vi "Laser.vi"(8 "error in (no error)":errorcluster, 10 "Notifiers":T1, 11 "All Message Queue Cluster":T2) -> (0 "error out":errorcluster)   [LabVIEW 2017]
doc: "Ce VI est la partie visualisation du Laser"
uses:
  Lib QMH/AllMessageQueue Cluster.ctl
  Lib QMH/Message Cluster.ctl
  Lib Notifier/Notifier.ctl
  Laser UI data.ctl
  Laser config.ctl
  FGV Laser/Action Laser.ctl
  FGV Laser/FGV Laser Data.ctl
  PulsePickerValues.ctl
  Lib IHM Control/Front Panel Status.ctl
  support/Status.vi
  Lib QMH/MessageQueues.lvlib
  Lib IHM Control/IHM Control.lvlib
  Lib Notifier/Notifier.lvlib
panel:
  out "AOM Freq":dbl format="%#_3g"
  out "Amp Freq":dbl format="%#_3g"
  out "Connected":bool
  out "Status":string
  # "Laser"
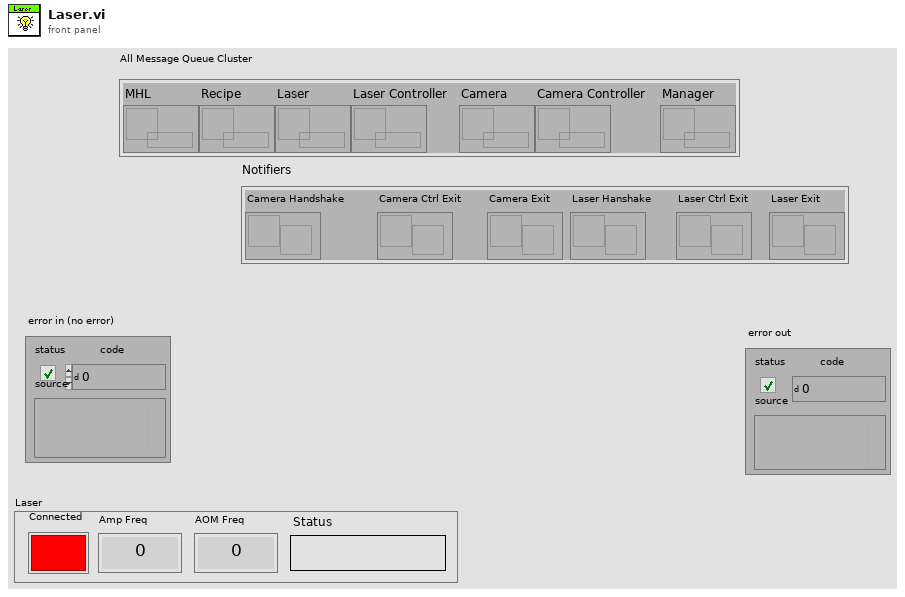
[diagram p1: front panel]
types:
  T1 = typedef "Notifier.lvlib/Notifier.ctl" = cluster{"Camera Handshake":refnum<notifier>, "Camera Ctrl Exit":refnum<notifier>, "Camera Exit":refnum<notifier>, "Laser Hanshake":refnum<notifier>, "Laser Ctrl Exit":refnum<notifier>, "Laser Exit":refnum<notifier>}
  T2 = typedef "MessageQueues.lvlib/AllMessageQueue Cluster.ctl" = cluster{"MHL":refnum<queue>, "Recipe":refnum<queue>, "Laser":refnum<queue>, "Laser Controller":refnum<queue>, "Camera":refnum<queue>, "Camera Controller":refnum<queue>, "Manager":refnum<queue>}
  T3 = typedef "FGV Laser Data.ctl" = cluster{"ONLINE":bool, "Power":dbl, "VISA resource name out":refnum<visa-resource-name>, "Time Out":dbl, "Status":string, "Read Count":u32, "On/OFF":bool, "Pulse Picker Set":T4}
  T4 = typedef "PulsePickerValues.ctl" = u16
  T5 = typedef "Action Laser.ctl" = enum16{"Initialize", "Connect", "Disconnect", "Set Power", "Get Power", "Set Pulse Picker", "Get Pulse Picker", "Laser ON", "Laser OFF", "Read Visa"}
  T6 = typedef "IHM Control.lvlib/Front Panel Status.ctl" = enum16{"Initialisation", "Enable Laser", "Enable Camera", "Disable Laser", "Disable Camera"}
  T7 = typedef "Laser config.ctl" = cluster{"VISA resource name":refnum<visa-resource-name>}
  T8 = typedef "Laser UI data.ctl" = cluster{"Connected":bool, "Status":string, "Power":dbl, "Pulse Picker":i32}
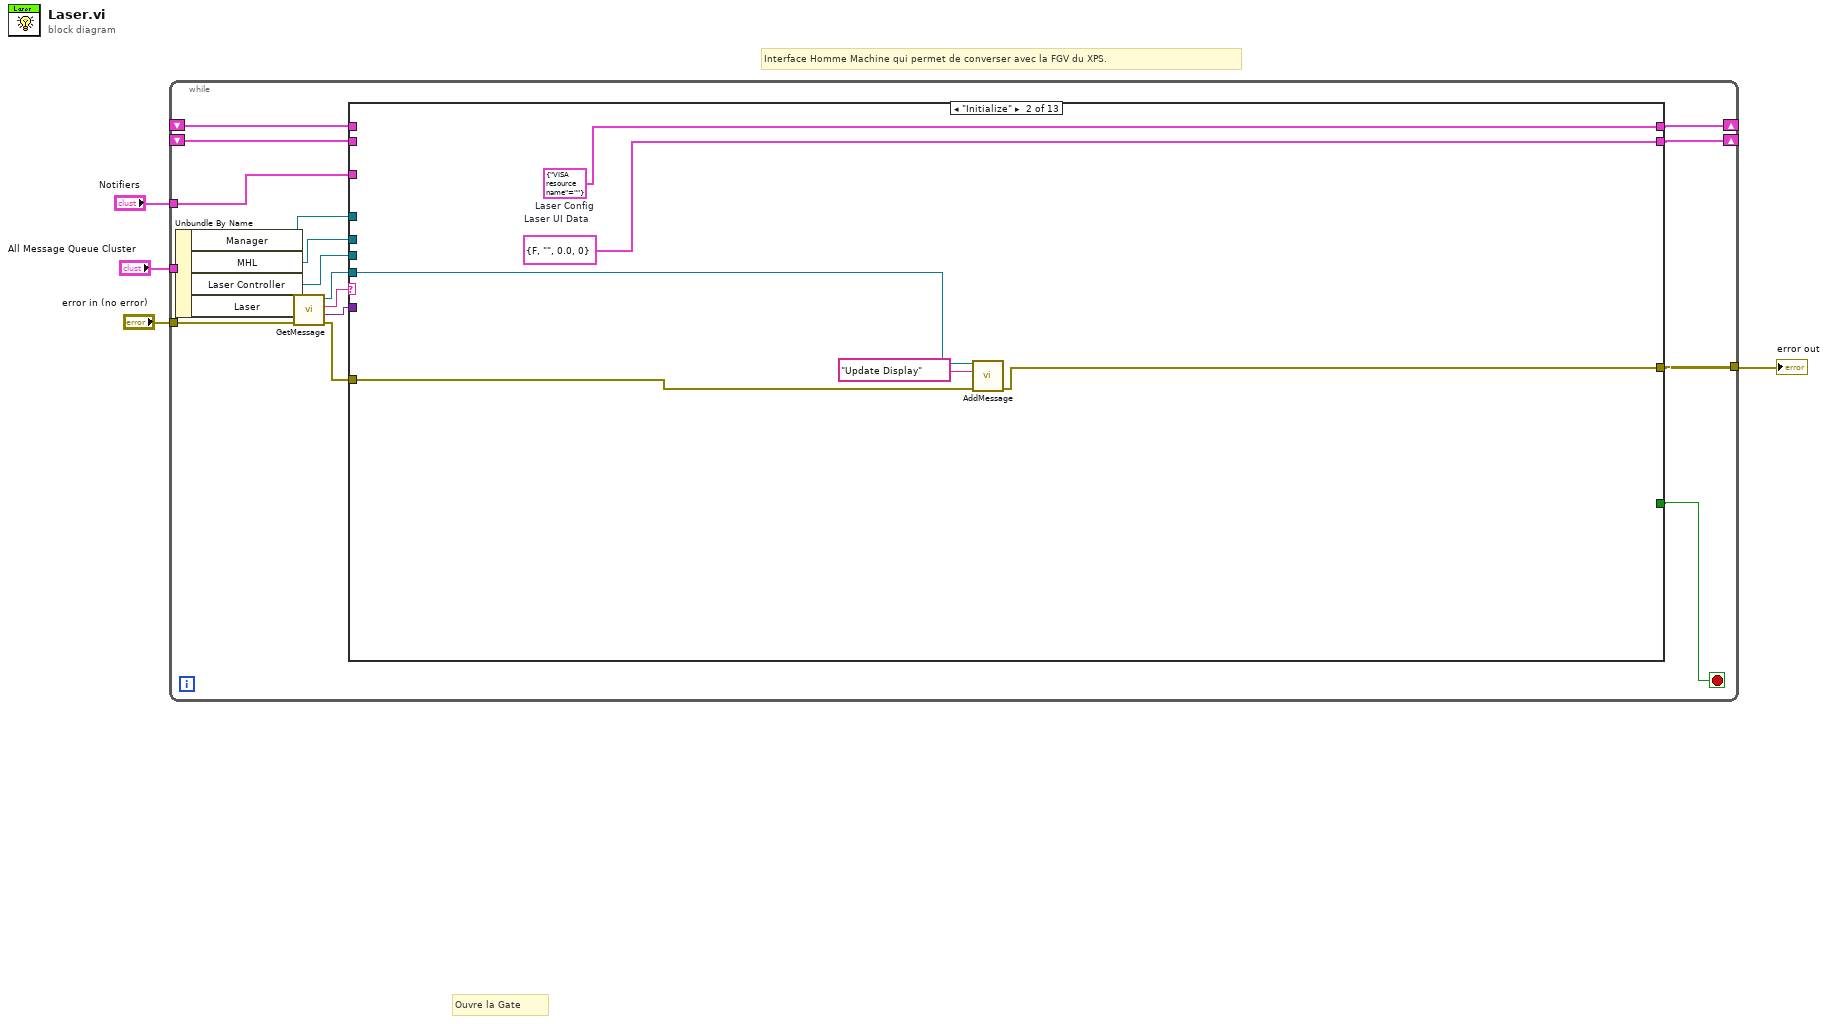
[diagram p0: block diagram]
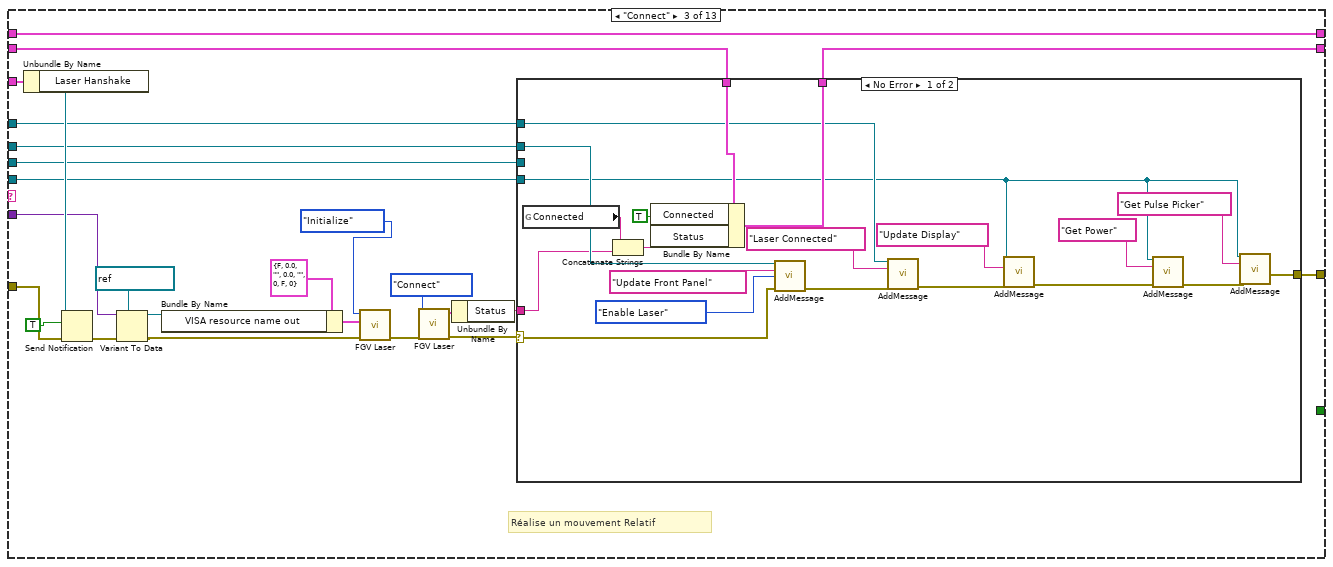
[diagram p3: hidden frame]
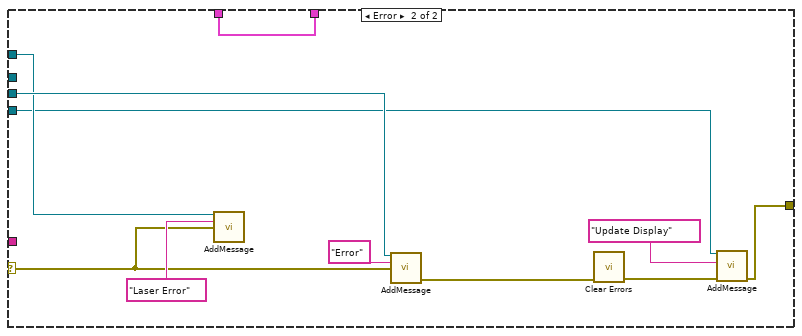
[diagram p4: hidden frame]
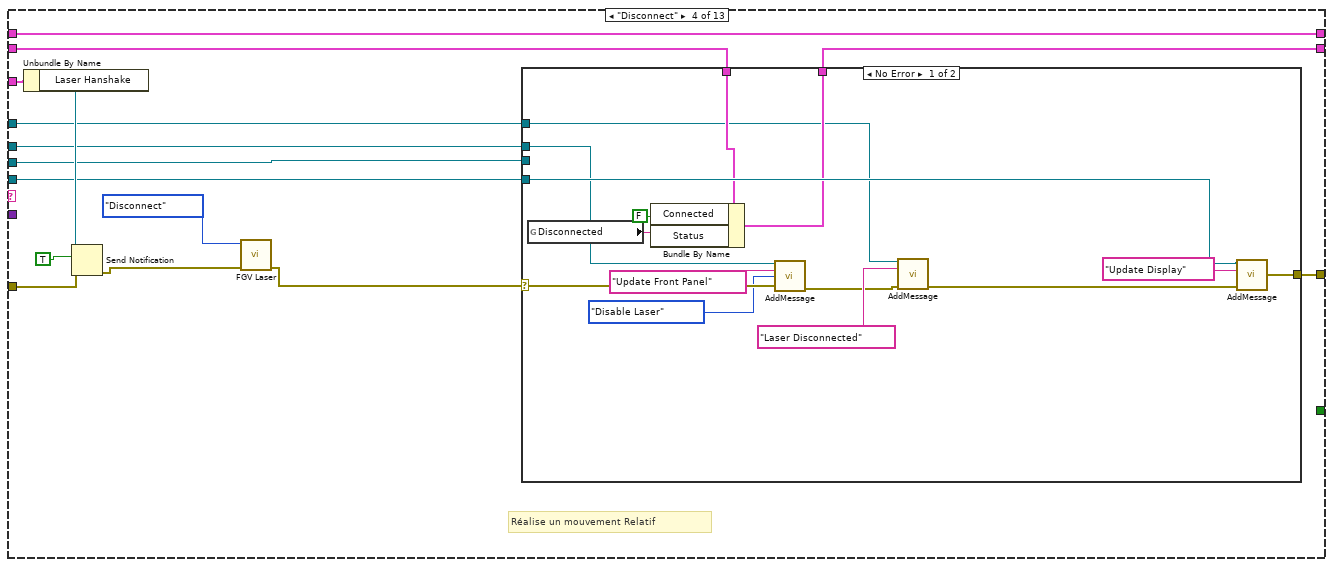
[diagram p5: hidden frame]
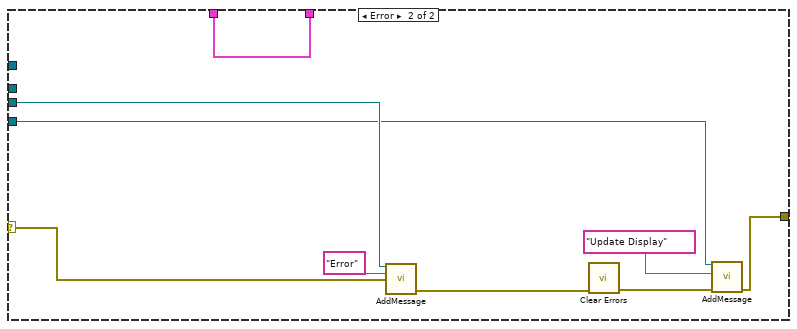
[diagram p6: hidden frame]
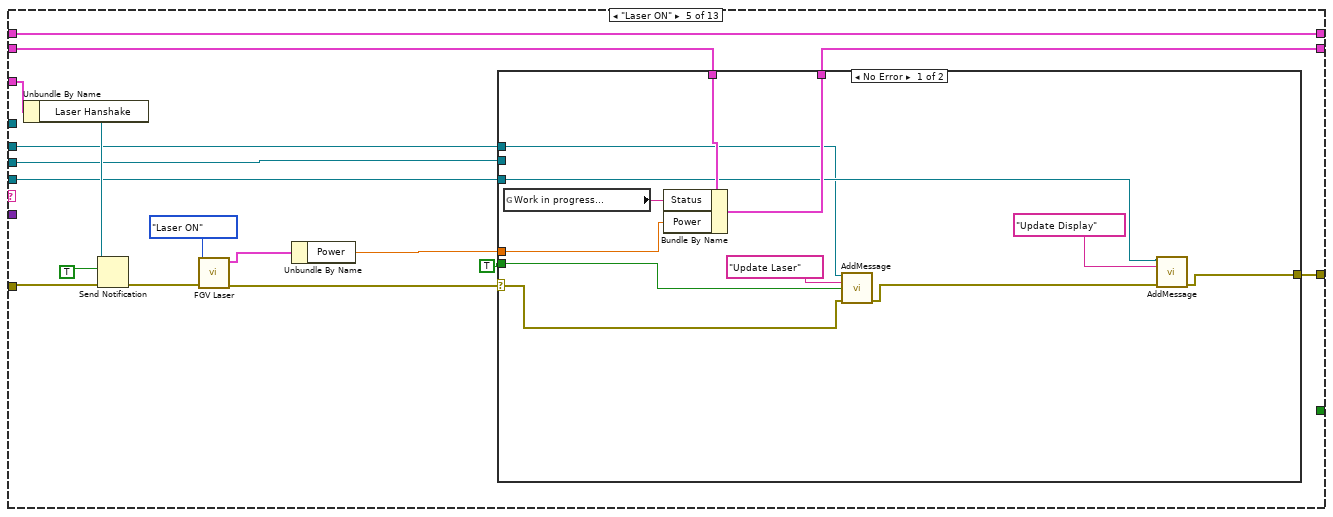
[diagram p7: hidden frame]
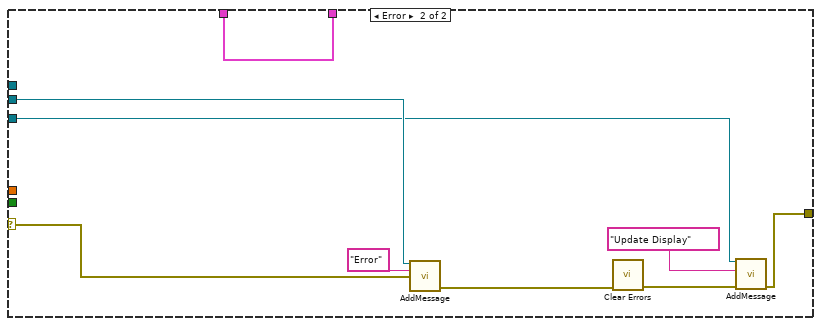
[diagram p8: hidden frame]
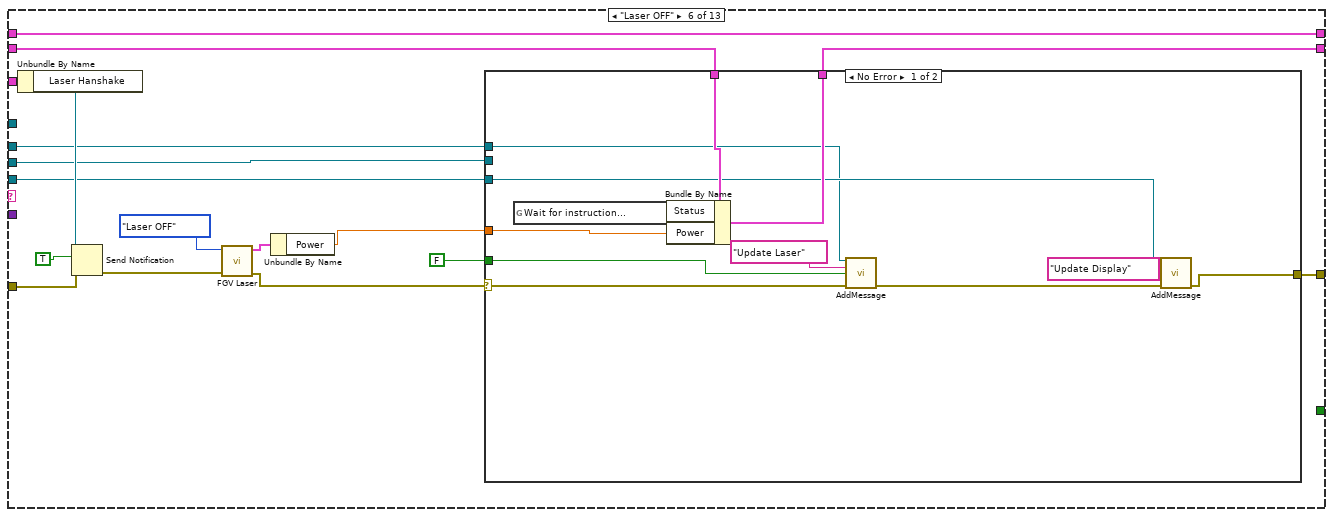
[diagram p9: hidden frame]
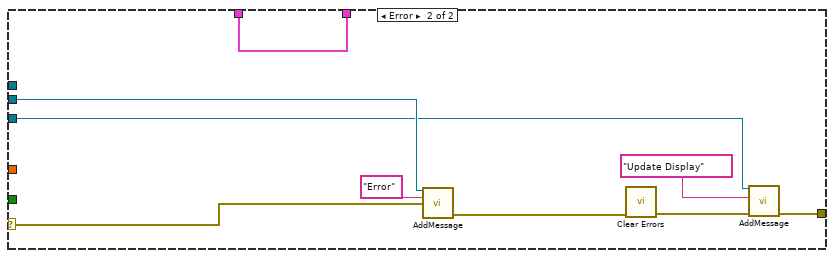
[diagram p10: hidden frame]
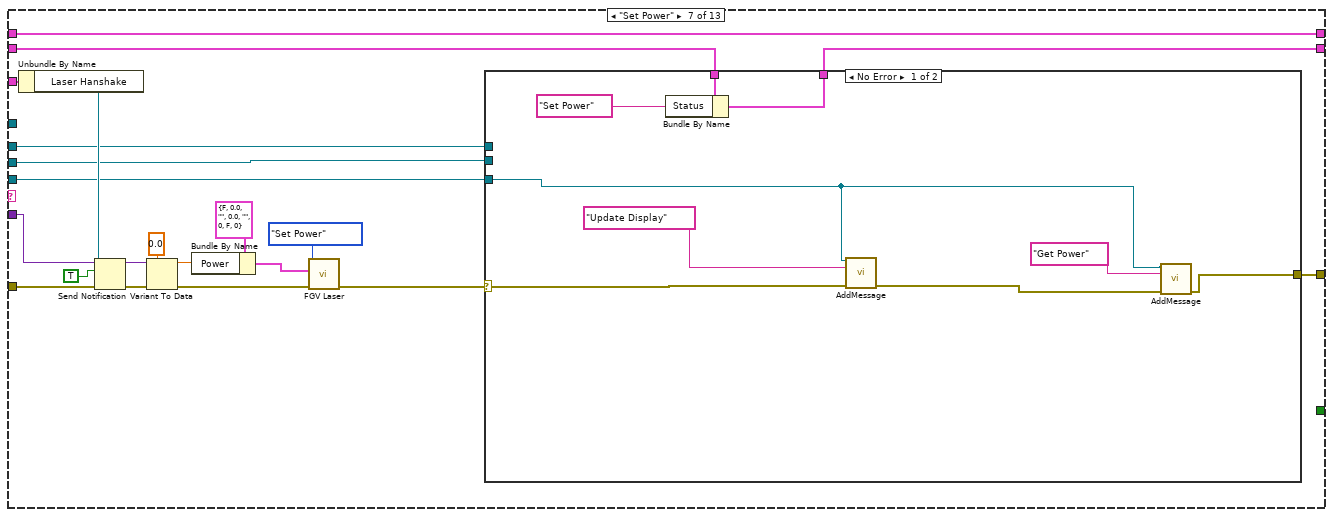
[diagram p11: hidden frame]
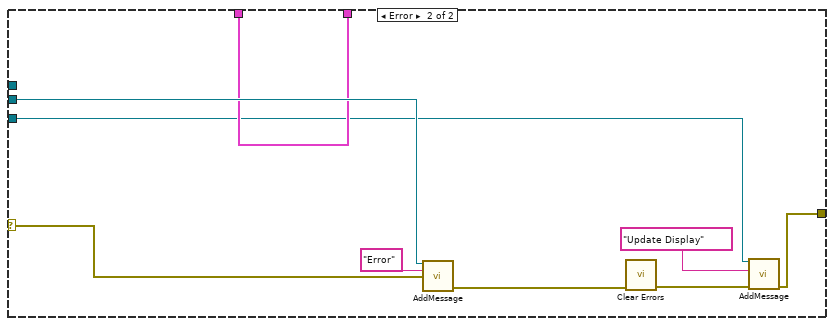
[diagram p12: hidden frame]
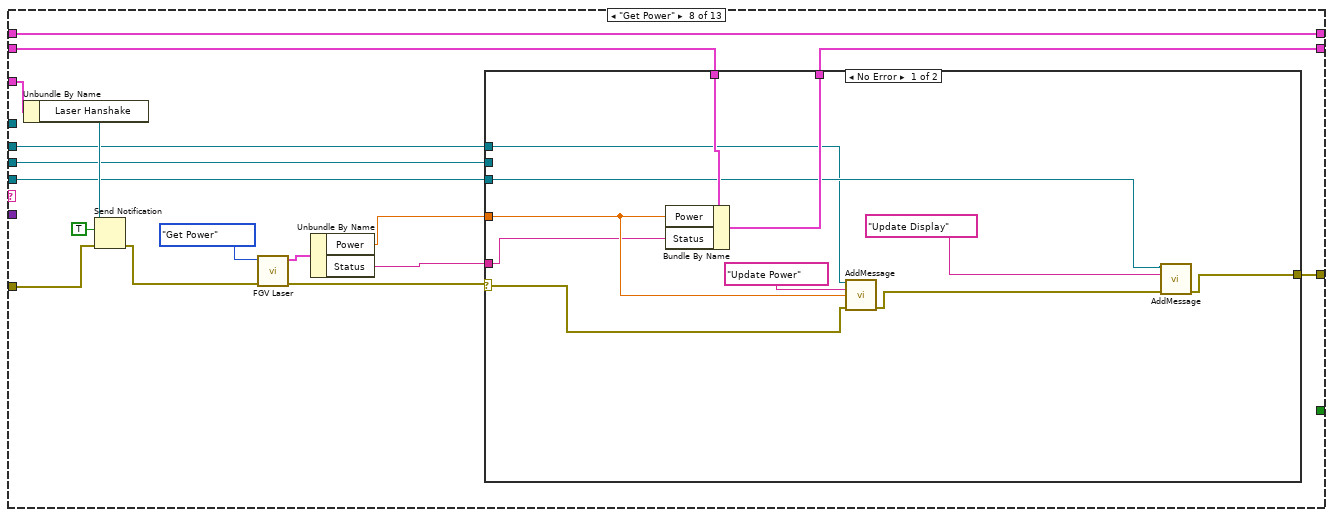
[diagram p13: hidden frame]
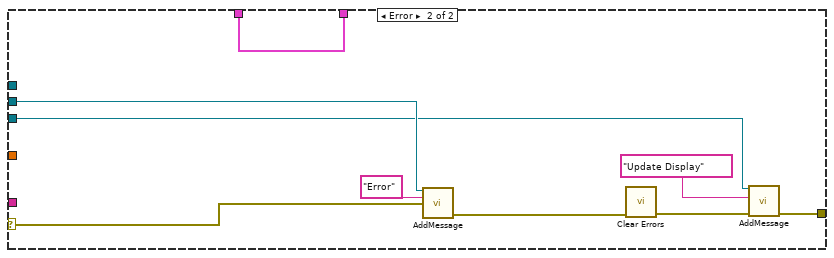
[diagram p14: hidden frame]
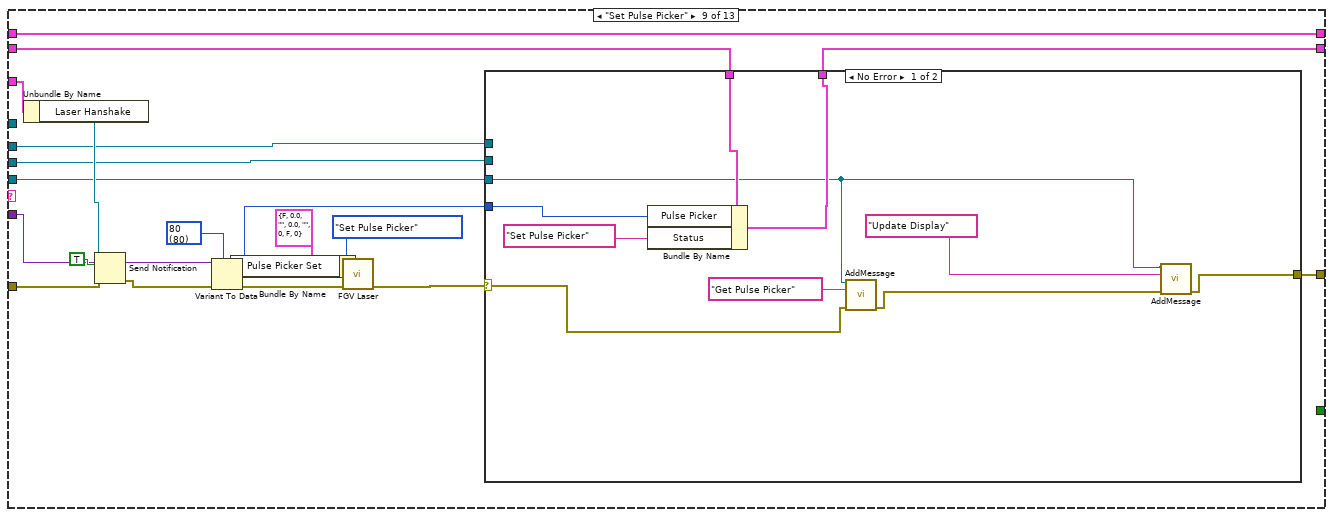
[diagram p15: hidden frame]
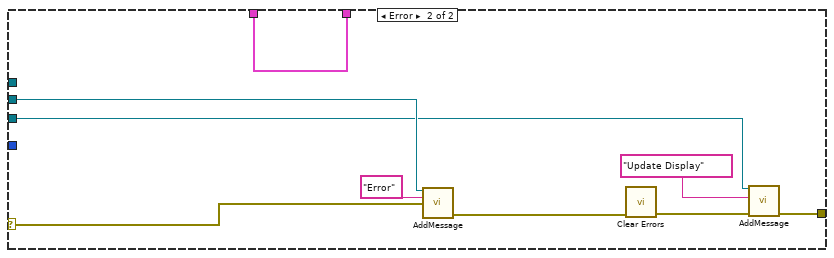
[diagram p16: hidden frame]
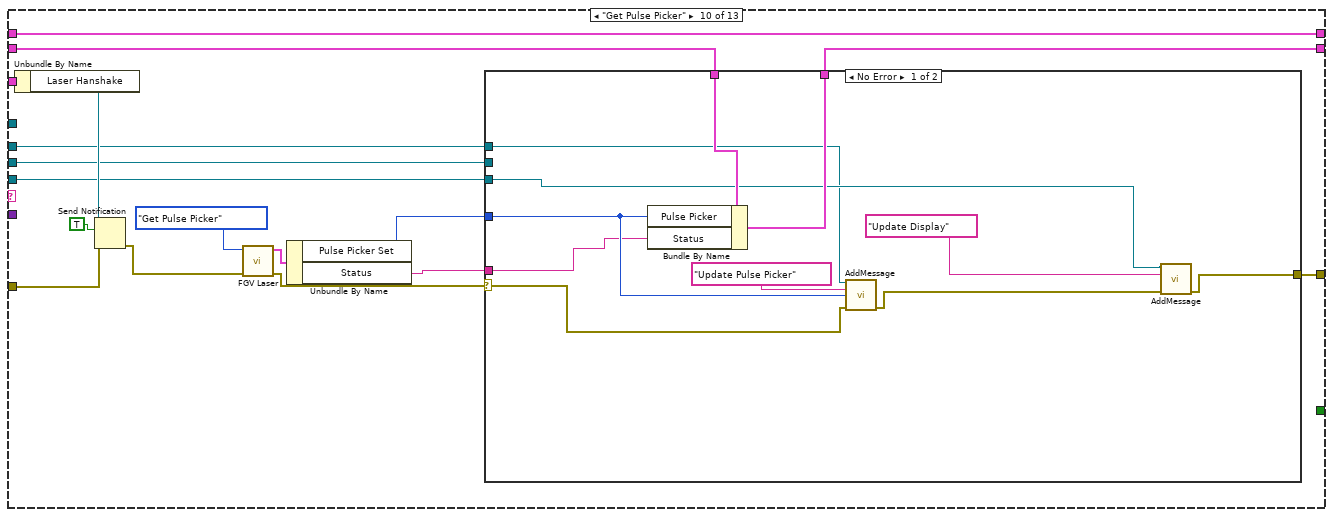
[diagram p17: hidden frame]
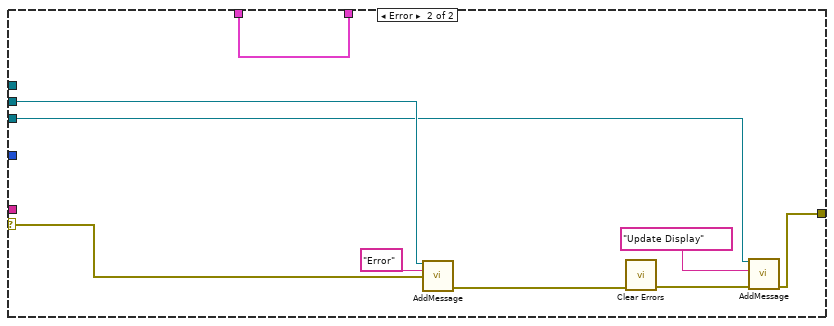
[diagram p18: hidden frame]
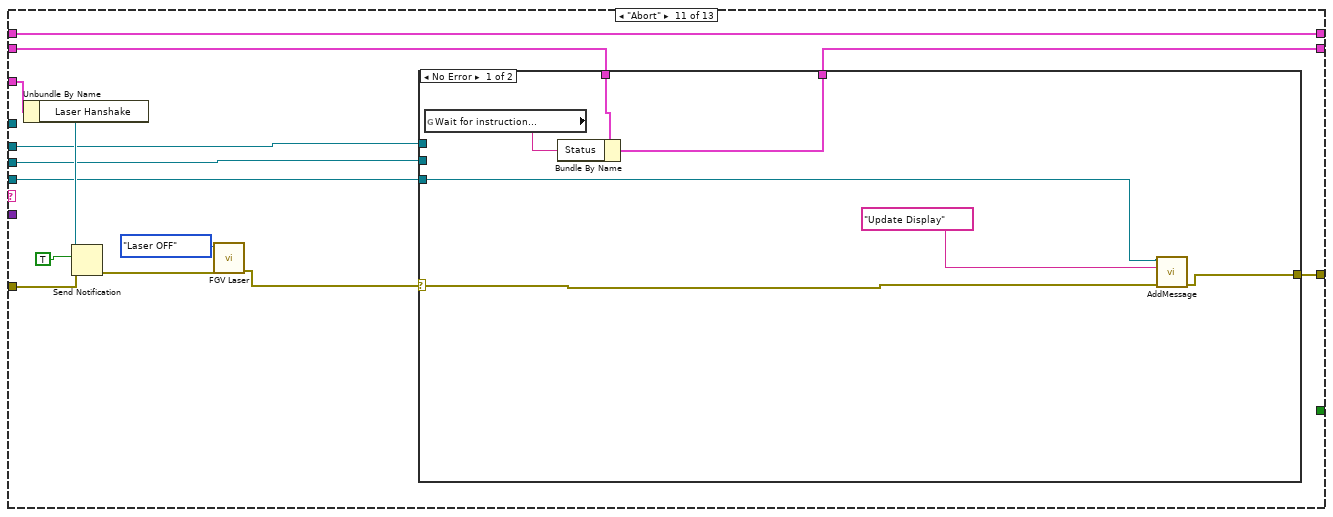
[diagram p19: hidden frame]
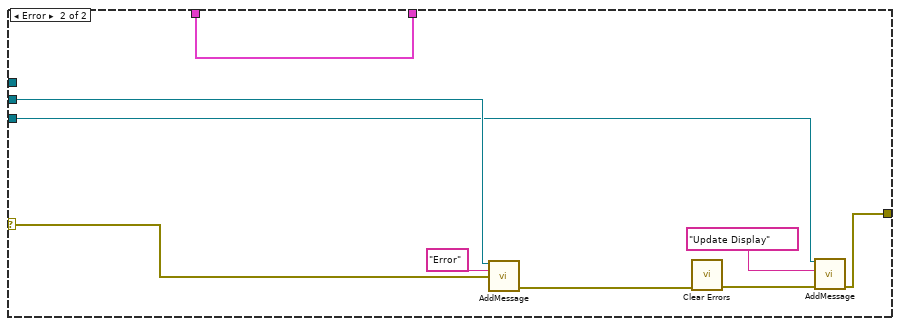
[diagram p20: hidden frame]
diagram:
  # "Interface Homme Machine qui permet de converser avec la FGV du XPS."
  # "Ouvre la Gate"
  n1 = while {
    tunnel: "All Message Queue Cluster" -> [w19]
    tunnel: "Notifiers" -> [w12]
    tunnel: "error in (no error)" -> [w20]
    tunnel: [w14] -> w1
    shift-right: [w16] -> _
    shift-left: _ -> [w18]
    shift-right: [w15] -> _
    shift-left: _ -> [w17]
    stop <- w13 stop-if-true
    n2 = Unbundle By Name(w19) -> ("Manager"=w11:refnum<queue>, "MHL"=w10:refnum<queue>, "Laser Controller"=w9:refnum<queue>, "Laser"=w21:refnum<queue>)
    n3 = call "GetMessage.vi"("entrée d'erreur"=w20, "Message queue"=w21) -> ("sortie d'erreur"=w7:errorcluster, "Data"=w6:variant, "Message"=w5:string, "Dup Message Queue"=w8:refnum<queue>)  [unwired: 6 in]
    n4 = case shown="\"Initialize\"" w5 {
      tunnel: w12 -> [_ _ w53 w100 w141 w179 w220 w255 w295 w331 w365 _ w400]
      tunnel: w8 -> [_ w27 w52 w99 w140 w178 w219 w254 w294 w330 w364 _ w394]
      tunnel: w6 -> [_ _ w42 _ _ _ w212 _ w287 _ _ _ _]
      tunnel: w7 -> [w24 w29 w46 w93 w135 w173 w210 w247 w286 w323 w359 w389 w395]
      tunnel: [w24 w28 w51 w98 w139 w177 w218 w253 w293 w329 w363 w389 w397] -> w14
      tunnel: w9 -> [_ _ w50 w97 w138 w176 w217 w252 w292 w328 w362 _ _]
      tunnel: [_ _ _ _ _ _ _ _ _ _ _ _ TRUE] -> w13
      tunnel: w18 -> [w23 _ w49 w96 w137 w175 w216 w251 w291 w327 w361 w390 w396]
      tunnel: [w23 w26 w49 w96 w137 w175 w216 w251 w291 w327 w361 w390 w396] -> w16
      tunnel: w17 -> [w22 _ w48 w95 w133 w171 w213 w248 w288 w324 w357 w388 w393]
      tunnel: [w22 w25 w47 w94 w136 w174 w215 w250 w290 w326 w360 w388 w393] -> w15
      tunnel: w10 -> [_ _ w45 w92 w134 w172 w214 w249 w289 w325 w358 _ _]
      tunnel: w11 -> [_ _ w44 w91 _ _ _ _ _ _ _ _ _]
      frame Default {
        # "ne fait rien si le message dépilé n'existe pas"
      }
      frame "Initialize" {
        w26 = T7 {"VISA resource name"=""}  # Laser Config
        w25 = T8 {"Connected"=FALSE, "Status"="", "Power"=0.0, "Pulse Picker"=0}  # Laser UI Data
        n5 = call "AddMessage.vi"("Message queue"=w27, "Message"="Update Display", "entrée d'erreur (pas d'erreur)"=w29) -> ("error out"=w28:errorcluster)  [unwired: 11 in, 1 out]
      }
      frame "Connect" {
        # "Réalise un mouvement Relatif"
        n6 = Unbundle By Name(w53) -> ("Laser Hanshake"=w55:refnum<notifier>)
        n7 = Send Notification(notification=TRUE, notifier=w55, error in (no error)=w46) -> (error out=w43:errorcluster)  [unwired: 1 out]
        n8 = Variant To Data(error in=w43, type=refnum<visa-resource-name> "COM30" ("VISA resource name out"), Variant=w42) -> (data=w36:refnum<visa-resource-name>, error out=w35:errorcluster)
        n9 = Bundle By Name(cluster=T3 {"ONLINE"=FALSE, "Power"=0.0, "VISA resource name out"="", "Time Out"=0.0, "Status"="", "Read Count"=0, "On/OFF"=FALSE, "Pulse Picker Set"=0} ("FGV Laser Data In"), "VISA resource name out"=w36) -> (w37:T3)
        n10 = call "FGV Laser.vi"("error in (no error)"=w35, "FGV Laser Data In"=w37, "Action"=Action_Laser."Initialize") -> ("error out"=w39:errorcluster)  [unwired: 7 in, 1 out]
        n11 = call "FGV Laser.vi"("error in (no error)"=w39, "Action"=Action_Laser."Connect") -> ("error out"=w33:errorcluster, "FGV Laser Data Out"=w32:T3)  [unwired: 8 in]
        n12 = Unbundle By Name(w32) -> ("Status"=w31:string)
        n13 = case shown="No Error" w33 {
          selector: w33 -> [w72 w78]
          tunnel: w52 -> [w57 w77]
          tunnel: [w59 w83] -> w51
          tunnel: w50 -> [_ w82]
          tunnel: w48 -> [w75 w81]
          tunnel: [w74 w81] -> w47
          tunnel: w45 -> [w71 _]
          tunnel: w44 -> [w66 w79]
          tunnel: w31 -> [w62 _]
          frame No Error {
            n14 = global read "Status.vi" "Connected"() -> (w64:string)
            n15 = Concatenate Strings(w64, w62) -> (w63:string)
            n16 = Bundle By Name(cluster=w75, "Connected"=TRUE, "Status"=w63) -> (w74:T8)
            n17 = call "AddMessage.vi"("Message queue"=w71, "Message"="Update Front Panel", "Data"=Front_Panel_Status."Enable Laser" ("Front Panel status"), "entrée d'erreur (pas d'erreur)"=w72) -> ("error out"=w68:errorcluster)  [unwired: 10 in, 1 out]
            n18 = call "AddMessage.vi"("Message queue"=w66, "Message"="Laser Connected", "entrée d'erreur (pas d'erreur)"=w68) -> ("error out"=w67:errorcluster)  [unwired: 11 in, 1 out]
            n19 = call "AddMessage.vi"("Message queue"=w57, "Message"="Update Display", "entrée d'erreur (pas d'erreur)"=w67) -> ("error out"=w61:errorcluster)  [unwired: 11 in, 1 out]
            n20 = call "AddMessage.vi"("Message queue"=w57, "Message"="Get Power", "entrée d'erreur (pas d'erreur)"=w61) -> ("error out"=w60:errorcluster)  [unwired: 11 in, 1 out]
            n21 = call "AddMessage.vi"("Message queue"=w57, "Message"="Get Pulse Picker", "entrée d'erreur (pas d'erreur)"=w60) -> ("error out"=w59:errorcluster)  [unwired: 11 in, 1 out]
          }
          frame Error {
            n22 = call "AddMessage.vi"("Message queue"=w79, "Message"="Laser Error", "Data"=w78) -> ()  [unwired: 11 in, 2 out]
            n23 = call "AddMessage.vi"("Message queue"=w82, "Message"="Error", "Data"=w78) -> ("error out"=w86:errorcluster)  [unwired: 11 in, 1 out]
            n24 = call <vilib>:"Clear Errors.vi"("error in (no error)"=w86) -> ("error out"=w84:errorcluster)  [unwired: 5 in, 1 out]
            n25 = call "AddMessage.vi"("Message queue"=w77, "Message"="Update Display", "entrée d'erreur (pas d'erreur)"=w84) -> ("error out"=w83:errorcluster)  [unwired: 11 in, 1 out]
          }
        }
      }
      frame "Disconnect" {
        # "Réalise un mouvement Relatif"
        n26 = Unbundle By Name(w100) -> ("Laser Hanshake"=w102:refnum<notifier>)
        n27 = Send Notification(notification=TRUE, notifier=w102, error in (no error)=w93) -> (error out=w90:errorcluster)  [unwired: 1 out]
        n28 = call "FGV Laser.vi"("error in (no error)"=w90, "Action"=Action_Laser."Disconnect") -> ("error out"=w89:errorcluster)  [unwired: 8 in, 1 out]
        n29 = case shown="No Error" w89 {
          selector: w89 -> [w111 w121]
          tunnel: w99 -> [w117 w118]
          tunnel: [w115 w122] -> w98
          tunnel: w97 -> [_ w120]
          tunnel: w95 -> [w114 w119]
          tunnel: [w113 w119] -> w94
          tunnel: w92 -> [w110 _]
          tunnel: w91 -> [w104 _]
          frame No Error {
            n30 = global read "Status.vi" "Disconnected"() -> (w103:string)
            n31 = Bundle By Name(cluster=w114, "Connected"=FALSE, "Status"=w103) -> (w113:T8)
            n32 = call "AddMessage.vi"("Message queue"=w110, "Message"="Update Front Panel", "Data"=Front_Panel_Status."Disable Laser" ("Front Panel status"), "entrée d'erreur (pas d'erreur)"=w111) -> ("error out"=w106:errorcluster)  [unwired: 10 in, 1 out]
            n33 = call "AddMessage.vi"("Message queue"=w104, "Message"="Laser Disconnected", "entrée d'erreur (pas d'erreur)"=w106) -> ("error out"=w105:errorcluster)  [unwired: 11 in, 1 out]
            n34 = call "AddMessage.vi"("Message queue"=w117, "Message"="Update Display", "entrée d'erreur (pas d'erreur)"=w105) -> ("error out"=w115:errorcluster)  [unwired: 11 in, 1 out]
          }
          frame Error {
            n35 = call "AddMessage.vi"("Message queue"=w120, "Message"="Error", "Data"=w121) -> ("error out"=w125:errorcluster)  [unwired: 11 in, 1 out]
            n36 = call <vilib>:"Clear Errors.vi"("error in (no error)"=w125) -> ("error out"=w123:errorcluster)  [unwired: 5 in, 1 out]
            n37 = call "AddMessage.vi"("Message queue"=w118, "Message"="Update Display", "entrée d'erreur (pas d'erreur)"=w123) -> ("error out"=w122:errorcluster)  [unwired: 11 in, 1 out]
          }
        }
      }
      frame "Laser ON" {
        n38 = Unbundle By Name(w141) -> ("Laser Hanshake"=w143:refnum<notifier>)
        n39 = Send Notification(notification=TRUE, notifier=w143, error in (no error)=w135) -> (error out=w131:errorcluster)  [unwired: 1 out]
        n40 = call "FGV Laser.vi"("error in (no error)"=w131, "Action"=Action_Laser."Laser ON") -> ("error out"=w130:errorcluster, "FGV Laser Data Out"=w128:T3)  [unwired: 8 in]
        n41 = Unbundle By Name(w128) -> ("Power"=w127:dbl)
        n42 = case shown="No Error" w130 {
          selector: w130 -> [w151 w159]
          tunnel: w140 -> [w152 w156]
          tunnel: [w146 w160] -> w139
          tunnel: w138 -> [_ w158]
          tunnel: w133 -> [w154 w157]
          tunnel: [w153 w157] -> w136
          tunnel: w134 -> [w149 _]
          tunnel: TRUE -> [w145 _]
          tunnel: w127 -> [w144 _]
          frame No Error {
            n43 = global read "Status.vi" "Work in progress..."() -> (w147:string)
            n44 = Bundle By Name(cluster=w154, "Status"=w147, "Power"=w144) -> (w153:T8)
            n45 = call "AddMessage.vi"("Message queue"=w149, "Message"="Update Laser", "Data"=w145, "entrée d'erreur (pas d'erreur)"=w151) -> ("error out"=w150:errorcluster)  [unwired: 10 in, 1 out]
            n46 = call "AddMessage.vi"("Message queue"=w152, "Message"="Update Display", "entrée d'erreur (pas d'erreur)"=w150) -> ("error out"=w146:errorcluster)  [unwired: 11 in, 1 out]
          }
          frame Error {
            n47 = call "AddMessage.vi"("Message queue"=w158, "Message"="Error", "Data"=w159) -> ("error out"=w163:errorcluster)  [unwired: 11 in, 1 out]
            n48 = call <vilib>:"Clear Errors.vi"("error in (no error)"=w163) -> ("error out"=w161:errorcluster)  [unwired: 5 in, 1 out]
            n49 = call "AddMessage.vi"("Message queue"=w156, "Message"="Update Display", "entrée d'erreur (pas d'erreur)"=w161) -> ("error out"=w160:errorcluster)  [unwired: 11 in, 1 out]
          }
        }
      }
      frame "Laser OFF" {
        n50 = Unbundle By Name(w179) -> ("Laser Hanshake"=w181:refnum<notifier>)
        n51 = Send Notification(notification=TRUE, notifier=w181, error in (no error)=w173) -> (error out=w169:errorcluster)  [unwired: 1 out]
        n52 = call "FGV Laser.vi"("error in (no error)"=w169, "Action"=Action_Laser."Laser OFF") -> ("error out"=w168:errorcluster, "FGV Laser Data Out"=w166:T3)  [unwired: 8 in]
        n53 = Unbundle By Name(w166) -> ("Power"=w165:dbl)
        n54 = case shown="No Error" w168 {
          selector: w168 -> [w183 w197]
          tunnel: w178 -> [w187 w194]
          tunnel: [w184 w198] -> w177
          tunnel: w176 -> [_ w196]
          tunnel: w171 -> [w189 w195]
          tunnel: [w188 w195] -> w174
          tunnel: w172 -> [w186 _]
          tunnel: FALSE -> [w185 _]
          tunnel: w165 -> [w182 _]
          frame No Error {
            n55 = global read "Status.vi" "Wait for instruction..."() -> (w190:string)
            n56 = Bundle By Name(cluster=w189, "Status"=w190, "Power"=w182) -> (w188:T8)
            n57 = call "AddMessage.vi"("Message queue"=w186, "Message"="Update Laser", "Data"=w185, "entrée d'erreur (pas d'erreur)"=w183) -> ("error out"=w192:errorcluster)  [unwired: 10 in, 1 out]
            n58 = call "AddMessage.vi"("Message queue"=w187, "Message"="Update Display", "entrée d'erreur (pas d'erreur)"=w192) -> ("error out"=w184:errorcluster)  [unwired: 11 in, 1 out]
          }
          frame Error {
            n59 = call "AddMessage.vi"("Message queue"=w196, "Message"="Error", "Data"=w197) -> ("error out"=w201:errorcluster)  [unwired: 11 in, 1 out]
            n60 = call <vilib>:"Clear Errors.vi"("error in (no error)"=w201) -> ("error out"=w199:errorcluster)  [unwired: 5 in, 1 out]
            n61 = call "AddMessage.vi"("Message queue"=w194, "Message"="Update Display", "entrée d'erreur (pas d'erreur)"=w199) -> ("error out"=w198:errorcluster)  [unwired: 11 in, 1 out]
          }
        }
      }
      frame "Set Power" {
        n62 = Unbundle By Name(w220) -> ("Laser Hanshake"=w222:refnum<notifier>)
        n63 = Send Notification(notification=TRUE, notifier=w222, error in (no error)=w210) -> (error out=w209:errorcluster)  [unwired: 1 out]
        n64 = Variant To Data(error in=w209, type=0.0, Variant=w212) -> (data=w207:dbl, error out=w205:errorcluster)
        n65 = Bundle By Name(cluster=T3 {"ONLINE"=FALSE, "Power"=0.0, "VISA resource name out"="", "Time Out"=0.0, "Status"="", "Read Count"=0, "On/OFF"=FALSE, "Pulse Picker Set"=0} ("FGV Laser Data In"), "Power"=w207) -> (w206:T3)
        n66 = call "FGV Laser.vi"("error in (no error)"=w205, "FGV Laser Data In"=w206, "Action"=Action_Laser."Set Power") -> ("error out"=w204:errorcluster)  [unwired: 7 in, 1 out]
        n67 = case shown="No Error" w204 {
          selector: w204 -> [w228 w235]
          tunnel: w219 -> [w225 w232]
          tunnel: [w227 w236] -> w218
          tunnel: w217 -> [_ w234]
          tunnel: w213 -> [w230 w233]
          tunnel: [w229 w233] -> w215
          tunnel: w214 -> [_ _]
          frame No Error {
            n68 = Bundle By Name(cluster=w230, "Status"="Set Power") -> (w229:T8)
            n69 = call "AddMessage.vi"("Message queue"=w225, "Message"="Update Display", "entrée d'erreur (pas d'erreur)"=w228) -> ("error out"=w231:errorcluster)  [unwired: 11 in, 1 out]
            n70 = call "AddMessage.vi"("Message queue"=w225, "Message"="Get Power", "entrée d'erreur (pas d'erreur)"=w231) -> ("error out"=w227:errorcluster)  [unwired: 11 in, 1 out]
          }
          frame Error {
            n71 = call "AddMessage.vi"("Message queue"=w234, "Message"="Error", "Data"=w235) -> ("error out"=w239:errorcluster)  [unwired: 11 in, 1 out]
            n72 = call <vilib>:"Clear Errors.vi"("error in (no error)"=w239) -> ("error out"=w237:errorcluster)  [unwired: 5 in, 1 out]
            n73 = call "AddMessage.vi"("Message queue"=w232, "Message"="Update Display", "entrée d'erreur (pas d'erreur)"=w237) -> ("error out"=w236:errorcluster)  [unwired: 11 in, 1 out]
          }
        }
      }
      frame "Get Power" {
        n74 = Unbundle By Name(w255) -> ("Laser Hanshake"=w257:refnum<notifier>)
        n75 = Send Notification(notification=TRUE, notifier=w257, error in (no error)=w247) -> (error out=w246:errorcluster)  [unwired: 1 out]
        n76 = call "FGV Laser.vi"("error in (no error)"=w246, "Action"=Action_Laser."Get Power") -> ("error out"=w245:errorcluster, "FGV Laser Data Out"=w243:T3)  [unwired: 8 in]
        n77 = Unbundle By Name(w243) -> ("Power"=w242:dbl, "Status"=w241:string)
        n78 = case shown="No Error" w245 {
          selector: w245 -> [w263 w272]
          tunnel: w254 -> [w261 w269]
          tunnel: [w262 w273] -> w253
          tunnel: w252 -> [_ w271]
          tunnel: w248 -> [w265 w270]
          tunnel: [w264 w270] -> w250
          tunnel: w249 -> [w260 _]
          tunnel: w242 -> [w259 _]
          tunnel: w241 -> [w258 _]
          frame No Error {
            n79 = Bundle By Name(cluster=w265, "Power"=w259, "Status"=w258) -> (w264:T8)
            n80 = call "AddMessage.vi"("Message queue"=w260, "Message"="Update Power", "Data"=w259, "entrée d'erreur (pas d'erreur)"=w263) -> ("error out"=w267:errorcluster)  [unwired: 10 in, 1 out]
            n81 = call "AddMessage.vi"("Message queue"=w261, "Message"="Update Display", "entrée d'erreur (pas d'erreur)"=w267) -> ("error out"=w262:errorcluster)  [unwired: 11 in, 1 out]
          }
          frame Error {
            n82 = call "AddMessage.vi"("Message queue"=w271, "Message"="Error", "Data"=w272) -> ("error out"=w276:errorcluster)  [unwired: 11 in, 1 out]
            n83 = call <vilib>:"Clear Errors.vi"("error in (no error)"=w276) -> ("error out"=w274:errorcluster)  [unwired: 5 in, 1 out]
            n84 = call "AddMessage.vi"("Message queue"=w269, "Message"="Update Display", "entrée d'erreur (pas d'erreur)"=w274) -> ("error out"=w273:errorcluster)  [unwired: 11 in, 1 out]
          }
        }
      }
      frame "Set Pulse Picker" {
        w278 = u16 80 items=["80"=80, "40"=40, "20"=20] ("Pulse Picker Set")
        n85 = Unbundle By Name(w295) -> ("Laser Hanshake"=w297:refnum<notifier>)
        n86 = Send Notification(notification=TRUE, notifier=w297, error in (no error)=w286) -> (error out=w285:errorcluster)  [unwired: 1 out]
        n87 = Variant To Data(error in=w285, type=w278, Variant=w287) -> (data=w279:u16, error out=w284:errorcluster)
        n88 = Bundle By Name(cluster=T3 {"ONLINE"=FALSE, "Power"=0.0, "VISA resource name out"="", "Time Out"=0.0, "Status"="", "Read Count"=0, "On/OFF"=FALSE, "Pulse Picker Set"=0} ("FGV Laser Data In"), "Pulse Picker Set"=w279) -> (w281:T3)
        n89 = call "FGV Laser.vi"("error in (no error)"=w284, "FGV Laser Data In"=w281, "Action"=Action_Laser."Set Pulse Picker") -> ("error out"=w283:errorcluster)  [unwired: 7 in, 1 out]
        n90 = case shown="No Error" w283 {
          selector: w283 -> [w302 w311]
          tunnel: w294 -> [w299 w308]
          tunnel: [w301 w312] -> w293
          tunnel: w292 -> [_ w310]
          tunnel: w288 -> [w304 w309]
          tunnel: [w303 w309] -> w290
          tunnel: w289 -> [_ _]
          tunnel: w279 -> [w298 _]
          frame No Error {
            n91 = Bundle By Name(cluster=w304, "Pulse Picker"=w298, "Status"="Set Pulse Picker") -> (w303:T8)
            n92 = call "AddMessage.vi"("Message queue"=w299, "Message"="Get Pulse Picker", "entrée d'erreur (pas d'erreur)"=w302) -> ("error out"=w306:errorcluster)  [unwired: 11 in, 1 out]
            n93 = call "AddMessage.vi"("Message queue"=w299, "Message"="Update Display", "entrée d'erreur (pas d'erreur)"=w306) -> ("error out"=w301:errorcluster)  [unwired: 11 in, 1 out]
          }
          frame Error {
            n94 = call "AddMessage.vi"("Message queue"=w310, "Message"="Error", "Data"=w311) -> ("error out"=w315:errorcluster)  [unwired: 11 in, 1 out]
            n95 = call <vilib>:"Clear Errors.vi"("error in (no error)"=w315) -> ("error out"=w313:errorcluster)  [unwired: 5 in, 1 out]
            n96 = call "AddMessage.vi"("Message queue"=w308, "Message"="Update Display", "entrée d'erreur (pas d'erreur)"=w313) -> ("error out"=w312:errorcluster)  [unwired: 11 in, 1 out]
          }
        }
      }
      frame "Get Pulse Picker" {
        n97 = Unbundle By Name(w331) -> ("Laser Hanshake"=w333:refnum<notifier>)
        n98 = Send Notification(notification=TRUE, notifier=w333, error in (no error)=w323) -> (error out=w322:errorcluster)  [unwired: 1 out]
        n99 = call "FGV Laser.vi"("error in (no error)"=w322, "Action"=Action_Laser."Get Pulse Picker") -> ("error out"=w321:errorcluster, "FGV Laser Data Out"=w319:T3)  [unwired: 8 in]
        n100 = Unbundle By Name(w319) -> ("Pulse Picker Set"=w318:T4, "Status"=w317:string)
        n101 = case shown="No Error" w321 {
          selector: w321 -> [w339 w348]
          tunnel: w330 -> [w337 w345]
          tunnel: [w338 w349] -> w329
          tunnel: w328 -> [_ w347]
          tunnel: w324 -> [w341 w346]
          tunnel: [w340 w346] -> w326
          tunnel: w325 -> [w336 _]
          tunnel: w318 -> [w335 _]
          tunnel: w317 -> [w334 _]
          frame No Error {
            n102 = Bundle By Name(cluster=w341, "Pulse Picker"=w335, "Status"=w334) -> (w340:T8)
            n103 = call "AddMessage.vi"("Message queue"=w336, "Message"="Update Pulse Picker", "Data"=w335, "entrée d'erreur (pas d'erreur)"=w339) -> ("error out"=w343:errorcluster)  [unwired: 10 in, 1 out]
            n104 = call "AddMessage.vi"("Message queue"=w337, "Message"="Update Display", "entrée d'erreur (pas d'erreur)"=w343) -> ("error out"=w338:errorcluster)  [unwired: 11 in, 1 out]
          }
          frame Error {
            n105 = call "AddMessage.vi"("Message queue"=w347, "Message"="Error", "Data"=w348) -> ("error out"=w352:errorcluster)  [unwired: 11 in, 1 out]
            n106 = call <vilib>:"Clear Errors.vi"("error in (no error)"=w352) -> ("error out"=w350:errorcluster)  [unwired: 5 in, 1 out]
            n107 = call "AddMessage.vi"("Message queue"=w345, "Message"="Update Display", "entrée d'erreur (pas d'erreur)"=w350) -> ("error out"=w349:errorcluster)  [unwired: 11 in, 1 out]
          }
        }
      }
      frame "Abort" {
        n108 = Unbundle By Name(w365) -> ("Laser Hanshake"=w367:refnum<notifier>)
        n109 = Send Notification(notification=TRUE, notifier=w367, error in (no error)=w359) -> (error out=w356:errorcluster)  [unwired: 1 out]
        n110 = call "FGV Laser.vi"("error in (no error)"=w356, "Action"=Action_Laser."Laser OFF") -> ("error out"=w354:errorcluster)  [unwired: 8 in, 1 out]
        n111 = case shown="No Error" w354 {
          selector: w354 -> [w372 w378]
          tunnel: w364 -> [w373 w375]
          tunnel: [w371 w379] -> w363
          tunnel: w362 -> [_ w377]
          tunnel: w357 -> [w370 w376]
          tunnel: [w369 w376] -> w360
          tunnel: w358 -> [_ _]
          frame No Error {
            n112 = global read "Status.vi" "Wait for instruction..."() -> (w368:string)
            n113 = Bundle By Name(cluster=w370, "Status"=w368) -> (w369:T8)
            n114 = call "AddMessage.vi"("Message queue"=w373, "Message"="Update Display", "entrée d'erreur (pas d'erreur)"=w372) -> ("error out"=w371:errorcluster)  [unwired: 11 in, 1 out]
          }
          frame Error {
            n115 = call "AddMessage.vi"("Message queue"=w377, "Message"="Error", "Data"=w378) -> ("error out"=w382:errorcluster)  [unwired: 11 in, 1 out]
            n116 = call <vilib>:"Clear Errors.vi"("error in (no error)"=w382) -> ("error out"=w380:errorcluster)  [unwired: 5 in, 1 out]
            n117 = call "AddMessage.vi"("Message queue"=w375, "Message"="Update Display", "entrée d'erreur (pas d'erreur)"=w380) -> ("error out"=w379:errorcluster)  [unwired: 11 in, 1 out]
          }
        }
      }
      frame "Update Display" {
        # "Met à jour les valeur Init, Status et position"
        n118 = Unbundle By Name(w388) -> ("Connected"=→"Connected":bool, "Status"=→"Status":string, "Power"=→"Amp Freq":dbl, "Pulse Picker"=→"AOM Freq":i32)
      }
      frame "Exit" {
        n119 = Unbundle By Name(w400) -> ("Laser Exit"=w399:refnum<notifier>)
        n120 = Release Queue(queue=w394, error in (no error)=w395) -> (error out=w391:errorcluster)  [unwired: 1 in, 2 out]
        n121 = call <vilib>:"Clear Errors.vi"("error in (no error)"=w391) -> ("error out"=w392:errorcluster)  [unwired: 5 in, 1 out]
        n122 = Send Notification(notification=TRUE, notifier=w399, error in (no error)=w392) -> (error out=w397:errorcluster)  [unwired: 1 out]
      }
    }
  }
  "error out" <- w1
